vi "TVE - 2 - Cópia.vi"(1 "Angle reference":dbl[](array[numeric]), 2 "Angle measured":dbl[](array[numeric]), 3 "Voltage reference":dbl[](array[numeric]), 4 "Voltage measured":dbl[](array[numeric])) -> (0 "Array":dbl[](array[numeric]))   [LabVIEW 2019]
panel:
  out "r * e^(i*theta) 2":cdb[](array[numeric])
  out "r * e^(i*theta)":cdb[](array[numeric])
  # "TVE calculation"
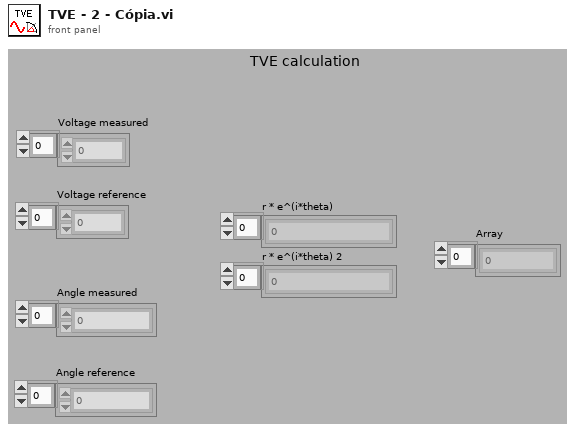
[diagram p1: front panel]
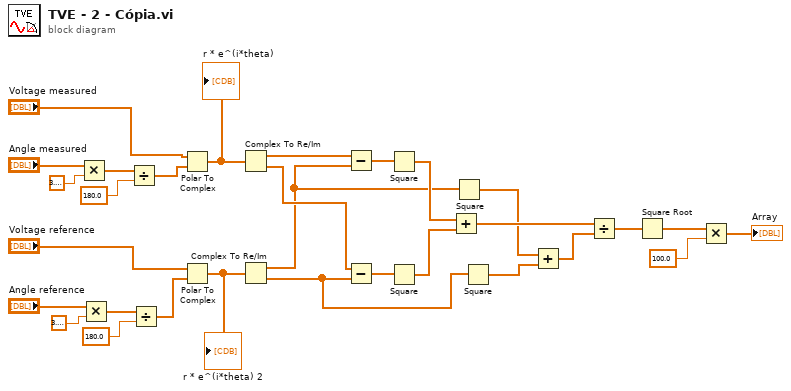
[diagram p0: block diagram]
diagram:
  n1 = Multiply(x="Angle measured", y=3.141592653589793) -> (x*y=w7:dbl[])
  n2 = Multiply(x="Angle reference", y=3.141592653589793) -> (x*y=w12:dbl[])
  n3 = Divide(x=w7, y=180.0) -> (x/y=w8:dbl[])
  n4 = Divide(x=w12, y=180.0) -> (x/y=w10:dbl[])
  n5 = Polar To Complex(1:w8, 2:"Voltage measured") -> (0:w19:cdb[])
  "r * e^(i*theta)" <- w19
  n6 = Polar To Complex(1:w10, 2:"Voltage reference") -> (0:w18:cdb[])
  "r * e^(i*theta) 2" <- w18
  n7 = Complex To Re/Im(x + iy=w19) -> (x=w17:dbl[], y=w16:dbl[])
  n8 = Complex To Re/Im(x + iy=w18) -> (x=w14:dbl[], y=w15:dbl[])
  n9 = Subtract(x=w17, y=w14) -> (x-y=w30:dbl[])
  n10 = Subtract(x=w16, y=w15) -> (x-y=w29:dbl[])
  n11 = Square(x=w30) -> (x^2=w21:dbl[])
  n12 = Square(x=w29) -> (x^2=w20:dbl[])
  n13 = Add(x=w21, y=w20) -> (x+y=w28:dbl[])
  n14 = Square(x=w14) -> (x^2=w26:dbl[])
  n15 = Square(x=w15) -> (x^2=w27:dbl[])
  n16 = Add(x=w26, y=w27) -> (x+y=w25:dbl[])
  n17 = Divide(x=w28, y=w25) -> (x/y=w24:dbl[])
  n18 = Square Root(x=w24) -> (sqrt(x)=w23:dbl[])
  n19 = Multiply(x=w23, y=100.0) -> (x*y=→"Array":dbl[])
